vi "swabian_initialize_stream.vi"(7 "acq_time":i64, 8 "error in (no error)":errorcluster, 10 "sync_rate 2":dbl, 11 "swabian_local_data":T1={"events"={"update_status"=refnum, "update_chart"=refnum, "update_xy"=refnum, "send_channel_data"=refnum}, "stop_q"=refnum, "tagger_reference"=refnum, "connect_button"=refnum, "counter_reference"=refnum, "tagger_stream_reference"=refnum, "log_reference"=refnum, "current_log_offset"=0, "tt20_buffer_q"=refnum, "stream_to_file_button"=refnum, "num_records"=0, "connected?"=FALSE, "plots"=refnum, "histogram_bin_edges"=[], "histogrammer"=refnum, "plot_lifetimes"=refnum, "xy_graph"=refnum, "Reference\nChannel"=enum."ch0", "trigger_channels"=[], "filter_channels"=[], "active_channels"=[], "acq_mode"=0, "Reference\nChannel"=enum."ch0", "acq_time"=0, "leftovers"={"leftover_stamps"=[], "leftover_channels"=[], "any?"=FALSE}, "sync_period_ps"=0, "raw_stream_path"=path "", "Leftovers"={"missing_sync_data"=[], "missing_events"=0}, "first_batch"=0, "first_sync_stamp"=0}) -> (0 "error out":errorcluster, 3 "swabian_local_data 2":T1={"events"={"update_status"=refnum, "update_chart"=refnum, "update_xy"=refnum, "send_channel_data"=refnum}, "stop_q"=refnum, "tagger_reference"=refnum, "connect_button"=refnum, "counter_reference"=refnum, "tagger_stream_reference"=refnum, "log_reference"=refnum, "current_log_offset"=0, "tt20_buffer_q"=refnum, "stream_to_file_button"=refnum, "num_records"=0, "connected?"=FALSE, "plots"=refnum, "histogram_bin_edges"=[], "histogrammer"=refnum, "plot_lifetimes"=refnum, "xy_graph"=refnum, "Reference\nChannel"=enum."ch0", "trigger_channels"=[], "filter_channels"=[], "active_channels"=[], "acq_mode"=0, "Reference\nChannel"=enum."ch0", "acq_time"=0, "leftovers"={"leftover_stamps"=[], "leftover_channels"=[], "any?"=FALSE}, "sync_period_ps"=0, "raw_stream_path"=path "", "Leftovers"={"missing_sync_data"=[], "missing_events"=0}, "first_batch"=0, "first_sync_stamp"=0})   [LabVIEW 2018]
uses:
  swabian_local_data_tdef.ctl
  swabian_events_tdef.ctl
  update_chart_tdef.ctl
  channel_data_tdef.ctl
  C:/Users/SWIR TCSPC/Desktop/Swabian/lib/TTCSharp32.dll
  lib/TTCSharp32.dll
  swabian_buffer_tdef.ctl
  reference_checkbox_tdef.ctl
  leftovers_struct.ctl
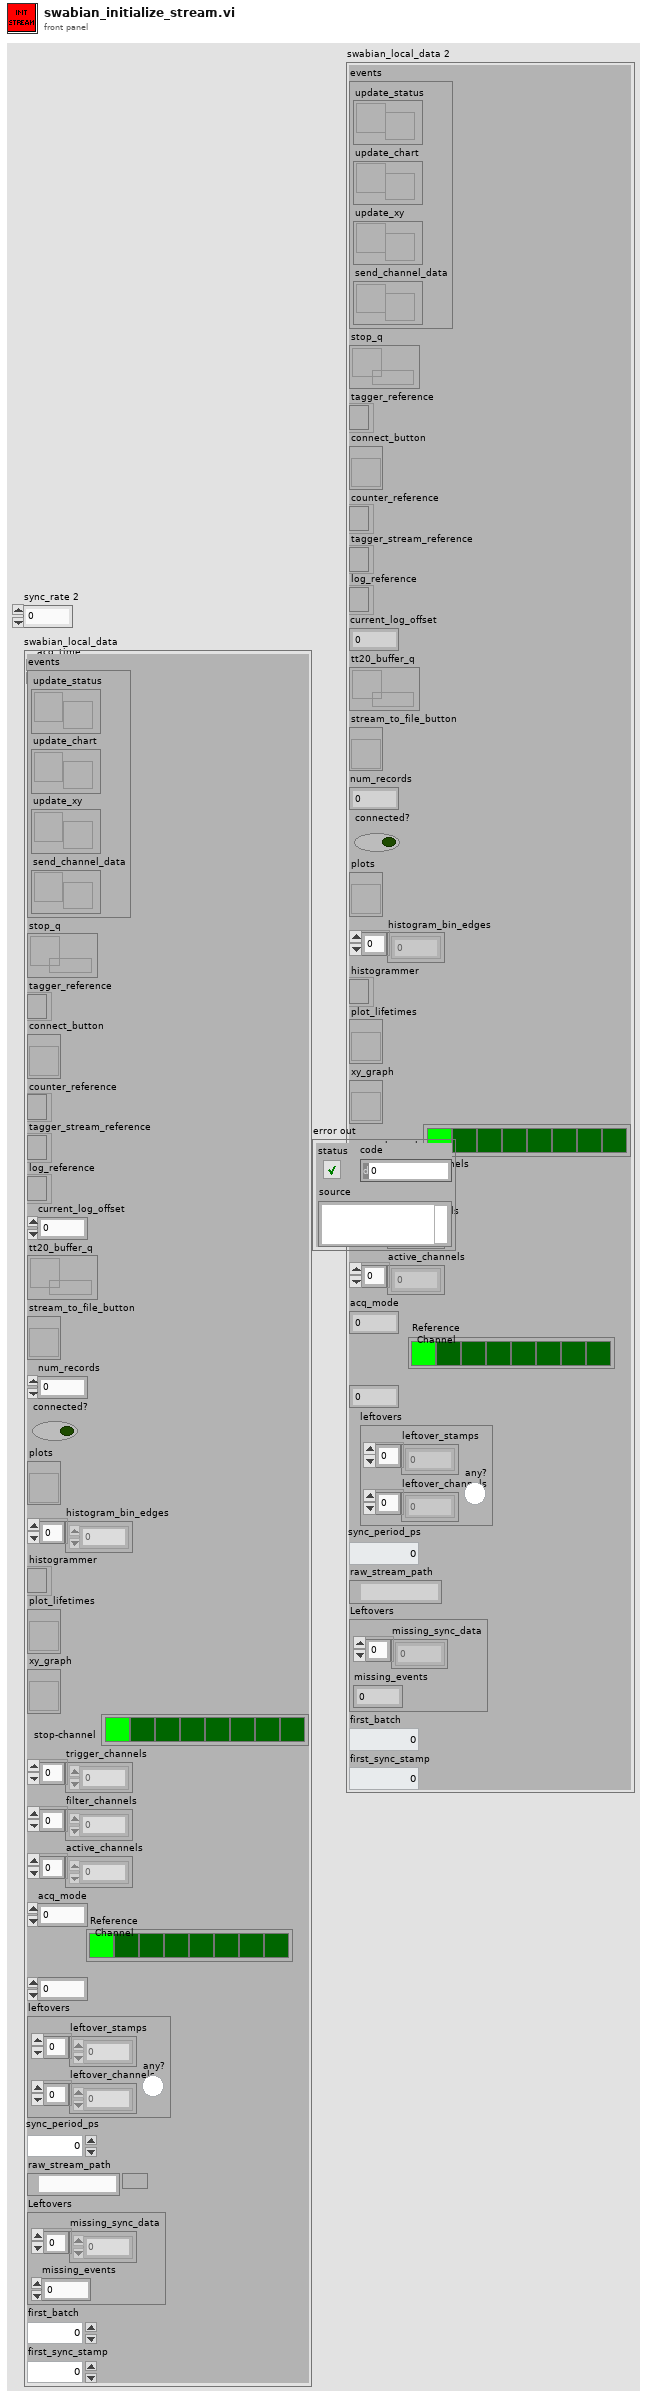
[diagram p1: front panel]
types:
  T1 = typedef "swabian_local_data_tdef.ctl" = cluster{"events":T2, "stop_q":refnum<queue>, "tagger_reference":refnum<k24>, "connect_button":refnum<vi>, "counter_reference":refnum<k24>, "tagger_stream_reference":refnum<k24>, "log_reference":refnum<file>, "current_log_offset":i64, "tt20_buffer_q":refnum<queue>, "stream_to_file_button":refnum<vi>, "num_records":u64, "connected?":bool, "plots":refnum<vi>, "histogram_bin_edges":i64[], "histogrammer":refnum<k24>, "plot_lifetimes":refnum<vi>, "xy_graph":refnum<vi>, "Reference\nChannel":T3, "trigger_channels":i32[], "filter_channels":i32[], "active_channels":i32[], "acq_mode":i32, "Reference\nChannel":T3, "acq_time":i64, "leftovers":T4, "sync_period_ps":i64, "raw_stream_path":path, "Leftovers":cluster{"missing_sync_data":u64[], "missing_events":i32}, "first_batch":i32, "first_sync_stamp":u64}
  T2 = typedef "swabian_events_tdef.ctl" = cluster{"update_status":refnum<user-event>, "update_chart":refnum<user-event>, "update_xy":refnum<user-event>, "send_channel_data":refnum<user-event>}
  T3 = typedef "reference_checkbox_tdef.ctl" = enum32{"No Selection", "ch0", "ch1", "ch2", "ch3", "ch4", "ch5", "ch6", "ch7"}
  T4 = typedef "leftovers_struct.ctl" = cluster{"leftover_stamps":i64[], "leftover_channels":i32[], "any?":bool}
  T5 = cluster{"missing_sync_data":u64[], "missing_events":i32}
  T6 = typedef "swabian_buffer_tdef.ctl" = cluster{"tagChannels":i32[], "tagTimestamps":i64[], "size":i32}
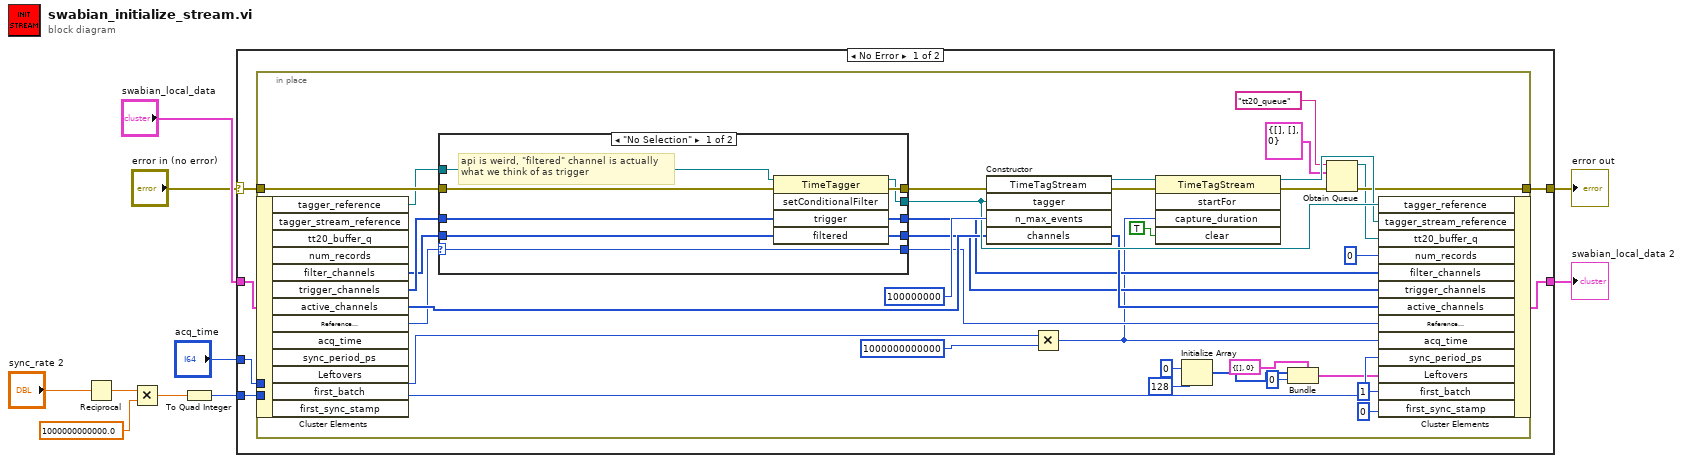
[diagram p0: block diagram]
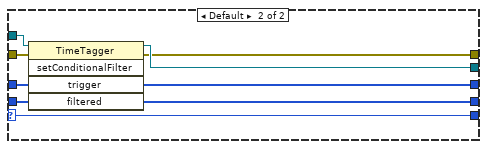
[diagram p2: hidden frame]
diagram:
  n1 = Reciprocal(x="sync_rate 2") -> (1/x=w4:dbl)
  n2 = Multiply(x=w4, y=1000000000000.0) -> (x*y=w2:dbl)
  n3 = To Quad Integer(1:w2) -> (0:w1:i64)
  n4 = case shown="No Error" "error in (no error)" {
    selector: "error in (no error)" -> [w12 w71]
    tunnel: "acq_time" -> [w16 _]
    tunnel: "swabian_local_data" -> [w15 w70]
    tunnel: [w14 w70] -> w8
    tunnel: [w13 w71] -> w7
    tunnel: w1 -> [w11 _]
    frame No Error {
      n5 = in-place {
        in-place-border: w12 -> [w37]
        in-place-border: w16 -> [w47]
        in-place-border: [w39] -> w13
        in-place-border: w11 -> [w25]
        n6 = in-place-cluster #1(w15) -> ("tagger_reference"=w36:refnum<k24>, "filter_channels"=w26:i32[], "trigger_channels"=w27:i32[], "active_channels"=w34:i32[], "Reference\nChannel"=w30:T3)  [unwired: 8 out]
        n7 = case shown="\"No Selection\"" w30 {
          selector: w30 -> [w54 w61]
          tunnel: w37 -> [w60 w66]
          tunnel: [w59 w67] -> w50
          tunnel: w36 -> [w58 w69]
          tunnel: [w57 w68] -> w44
          tunnel: w27 -> [w53 w65]
          tunnel: w26 -> [w52 w64]
          tunnel: [w56 w63] -> w32
          tunnel: [w55 w62] -> w31
          tunnel: [w54 w61] -> w29
          frame "No Selection" {
            # "api is weird, \"filtered\" channel is actually\nwhat we think of as trigger"
            n8 = invoke class="TimeTagger" method="setConditionalFilter"(reference=w58, error in=w60, "trigger"=w53, "filtered"=w52) -> (reference out=w57:refnum<k24>, error out=w59:errorcluster, "trigger"=w56:i32[], "filtered"=w55:i32[])  [unwired: 1 in, 1 out]
          }
          frame Default {
            n9 = invoke class="TimeTagger" method="setConditionalFilter"(reference=w69, error in=w66, "trigger"=w65, "filtered"=w64) -> (reference out=w68:refnum<k24>, error out=w67:errorcluster, "trigger"=w63:i32[], "filtered"=w62:i32[])  [unwired: 1 in, 1 out]
          }
        }
        n10 = constructor class="TimeTagStream"(error in=w50, "tagger"=w44, "n_max_events"=100000000, "channels"=w34) -> (reference out=w48:refnum<k24>, error out=w49:errorcluster, "channels"=w33:i32[])  [unwired: 2 in, 3 out]
        n11 = Multiply(x=w47, y=i64 1000000000000) -> (x*y=w28:i64)
        n12 = invoke class="TimeTagStream" method="startFor"(reference=w48, error in=w49, "capture_duration"=w28, "clear"=TRUE) -> (reference out=w43:refnum<k24>, error out=w40:errorcluster)  [unwired: 1 in, 3 out]
        n13 = Initialize Array(u64 0 ("element"), 128 ("dimension size")) -> (w21:u64[])
        n14 = Bundle(cluster=T5 {"missing_sync_data"=[], "missing_events"=0} ("Leftovers"), "missing_sync_data"=w21, "missing_events"=0) -> (w19:T5)
        n15 = Obtain Queue(name (unnamed)="tt20_queue", element data type=T6 {"tagChannels"=[], "tagTimestamps"=[], "size"=0} ("swabian_buffer"), error in (no error)=w40) -> (queue out=w38:refnum<queue>, error out=w39:errorcluster)  [unwired: 2 in, 1 out]
        n16 = in-place-cluster #1("tagger_reference"=w44, "tagger_stream_reference"=w43, "tt20_buffer_q"=w38, "num_records"=u64 0, "filter_channels"=w32, "trigger_channels"=w31, "active_channels"=w33, "Reference\nChannel"=w29, "acq_time"=w28, "sync_period_ps"=w25, "Leftovers"=w19, "first_batch"=1, "first_sync_stamp"=u64 0) -> (w14:T1)
      }
    }
    frame Error {
    }
  }
  "swabian_local_data 2" <- w8
  "error out" <- w7
